vi "Set_TempHumWindDir_Calibration.vi"(5 "Wind dir off":i32, 6 "Path":path, 7 "Outside hum":dbl, 8 "Inside hum.":dbl, 9 "Outside temp":dbl min=-7.0 max=7.0 step=0.01, 10 "Inside temp":dbl min=-7.0 max=7.0 step=0.01) -> (0 "Cor. out hum":dbl, 1 "Cor. in hum":dbl, 2 "Cor. out temp":dbl, 3 "Cor. in temp":dbl, 4 "Calibration values set?":bool)   [LabVIEW 2012]
uses:
  VantagePro.dll
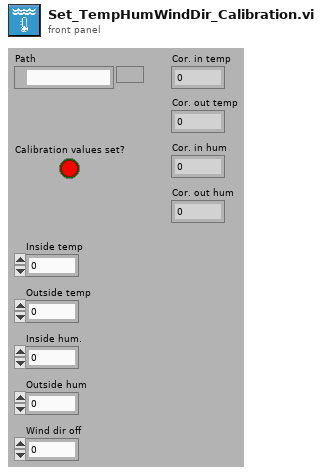
[diagram p1: front panel]
types:
  T1 = cluster{"In Temp":sgl, "Out Temp":sgl, "In Hum":u8, "Out Hum":u8, "Dum":i8, "Dum":i8, "Off In Temp":sgl, "Off Out Temp":sgl, "Off In Hum":i8, "Off Out Hum":i8}
  T2 = cluster{"In Temp":dbl, "Out Temp":dbl, "In Hum":dbl, "Out Hum":dbl}
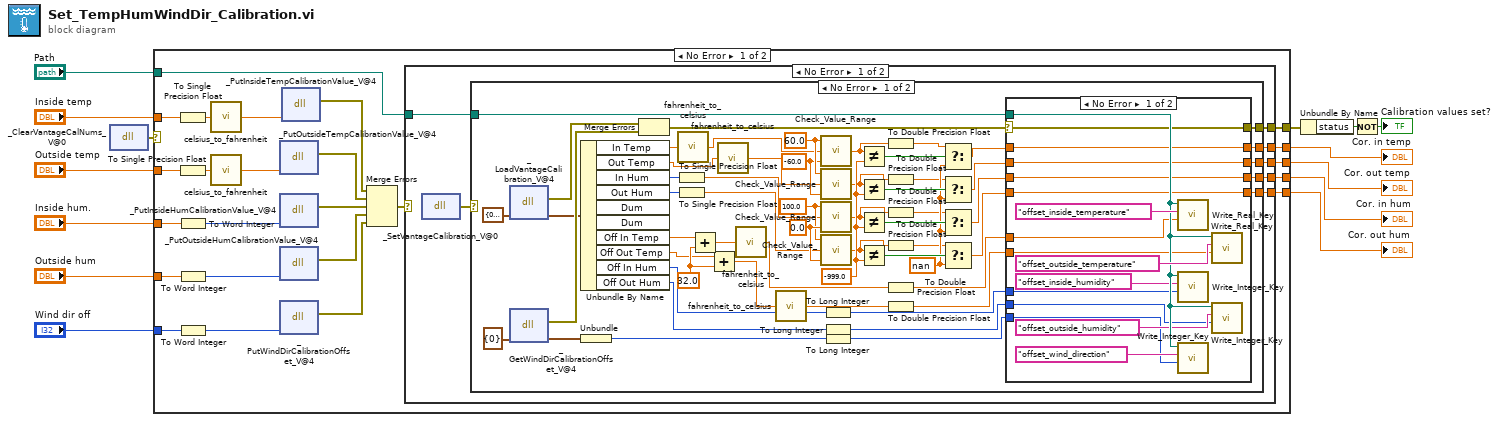
[diagram p0: block diagram]
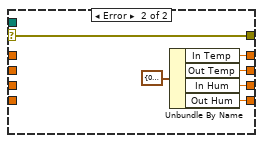
[diagram p2: hidden frame]
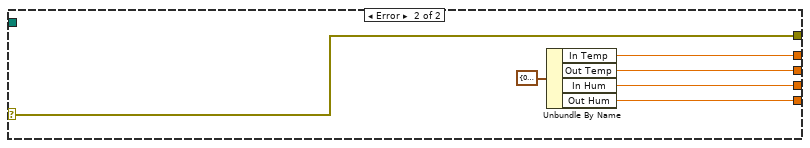
[diagram p3: hidden frame]
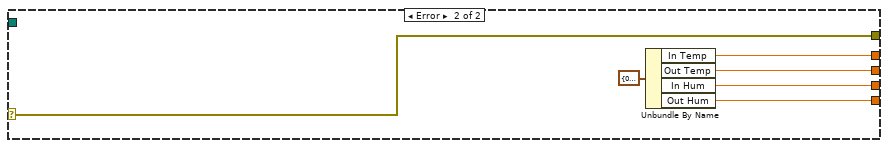
[diagram p4: hidden frame]
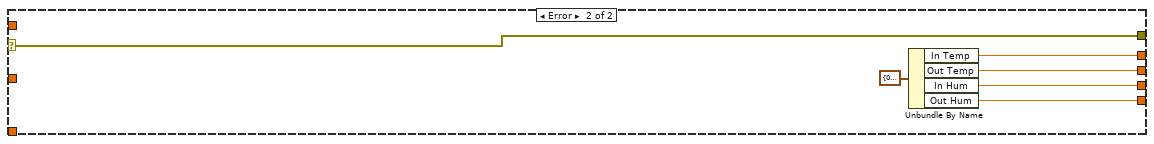
[diagram p5: hidden frame]
diagram:
  n1 = dll-call lib="C:/Users/Bob van Eijk/Desktop/LabView Projects 12/HiSPARC Weather Station/VantagePro.dll" fn="_ClearVantageCalNums_V@0" label="Clear Cal Nums"() -> (error out=w14:errorcluster)  [unwired: 4 in, 1 out]
  n2 = case shown="No Error" w14 {
    selector: w14 -> [_ w143]
    tunnel: "Inside temp" -> [w27 _]
    tunnel: "Inside hum." -> [w25 _]
    tunnel: "Outside temp" -> [w26 _]
    tunnel: "Outside hum" -> [w24 _]
    tunnel: "Wind dir off" -> [w23 _]
    tunnel: "Path" -> [w33 _]
    tunnel: [w32 w143] -> w7
    tunnel: [w31 w141] -> w4
    tunnel: [w30 w140] -> w3
    tunnel: [w29 w139] -> w2
    tunnel: [w28 w138] -> w1
    frame No Error {
      n3 = To Single Precision Float(number=w27) -> (single precision float=w35:sgl)
      n4 = To Single Precision Float(number=w26) -> (single precision float=w36:sgl)
      n5 = To Word Integer(number=w25) -> (16bit integer=w16:i16)
      n6 = To Word Integer(number=w24) -> (16bit integer=w15:i16)
      n7 = To Word Integer(number=w23) -> (16bit integer=w37:i16)
      n8 = call "celsius_to_fahrenheit.vi"("Celcius"=w35) -> ("Fahrenheit"=w22:sgl)
      n9 = call "celsius_to_fahrenheit.vi"("Celcius"=w36) -> ("Fahrenheit"=w17:sgl)
      n10 = dll-call lib="C:/Users/Bob van Eijk/Desktop/LabView Projects 12/HiSPARC Weather Station/VantagePro.dll" fn="_PutOutsideTempCalibrationValue_V@4" label="Put Out Temp Cal Val"("valValue"=w17) -> (error out=w20:errorcluster)  [unwired: 5 in, 1 out]
      n11 = dll-call lib="C:/Users/Bob van Eijk/Desktop/LabView Projects 12/HiSPARC Weather Station/VantagePro.dll" fn="_PutInsideHumCalibrationValue_V@4" label="Put In Hum Cal Val"("calValue"=w16) -> (error out=w19:errorcluster)  [unwired: 5 in, 1 out]
      n12 = dll-call lib="C:/Users/Bob van Eijk/Desktop/LabView Projects 12/HiSPARC Weather Station/VantagePro.dll" fn="_PutOutsideHumCalibrationValue_V@4" label="Put Out Hum Cal Val"("calValue"=w15) -> (error out=w18:errorcluster)  [unwired: 5 in, 1 out]
      n13 = dll-call lib="C:/Users/Bob van Eijk/Desktop/LabView Projects 12/HiSPARC Weather Station/VantagePro.dll" fn="_PutWindDirCalibrationOffset_V@4" label="Wind dir Offset"("winddirectionoff"=w37) -> (error out=w38:errorcluster)  [unwired: 5 in, 1 out]
      n14 = dll-call lib="C:/Users/Bob van Eijk/Desktop/LabView Projects 12/HiSPARC Weather Station/VantagePro.dll" fn="_PutInsideTempCalibrationValue_V@4" label="Put In Temp Cal Val"("calValue"=w22) -> (error out=w21:errorcluster)  [unwired: 5 in, 1 out]
      n15 = Merge Errors(w21, w20, w19, w18, w38) -> (w34:errorcluster)
      n16 = case shown="No Error" w34 {
        selector: w34 -> [_ w137]
        tunnel: [w43 w137] -> w32
        tunnel: w33 -> [w44 _]
        tunnel: [w42 w135] -> w31
        tunnel: [w41 w134] -> w30
        tunnel: [w40 w133] -> w29
        tunnel: [w39 w132] -> w28
        frame No Error {
          n17 = dll-call lib="C:/Users/Bob van Eijk/Desktop/LabView Projects 12/HiSPARC Weather Station/VantagePro.dll" fn="_SetVantageCalibration_V@0" label="Set cal. val."() -> (error out=w45:errorcluster)  [unwired: 4 in, 1 out]
          n18 = case shown="No Error" w45 {
            selector: w45 -> [_ w126]
            tunnel: [w81 w127] -> w39
            tunnel: [w82 w128] -> w40
            tunnel: [w83 w129] -> w41
            tunnel: [w84 w130] -> w42
            tunnel: [w79 w126] -> w43
            tunnel: w44 -> [w80 _]
            frame No Error {
              w59 = nan ("Data_input")
              w68 = sgl -999.0 ("Min")
              w78 = sgl 0.0 ("Min")
              w77 = sgl 100.0 ("Max")
              w75 = sgl -60.0 ("Min")
              w76 = sgl 60.0 ("Max")
              w96 = sgl 32.0
              n19 = dll-call lib="C:/Users/Bob van Eijk/Desktop/LabView Projects 12/HiSPARC Weather Station/VantagePro.dll" fn="_LoadVantageCalibration_V@4" label="Temp&hum data"("calibration"=T1 {"In Temp"=0.0, "Out Temp"=0.0, "In Hum"=0, "Out Hum"=0, "Dum"=0, "Dum"=0, "Off In Temp"=0.0, "Off Out Temp"=0.0, "Off In Hum"=0, "Off Out Hum"=0}) -> (error out=w100:errorcluster, "calibration"=w93:T1)  [unwired: 4 in, 1 out]
              n20 = dll-call lib="C:/Users/Bob van Eijk/Desktop/LabView Projects 12/HiSPARC Weather Station/VantagePro.dll" fn="_GetWindDirCalibrationOffset_V@4" label="Wind dir offset"("winddirectionoff"=cluster{i32} {0}) -> (error out=w101:errorcluster, "winddirectionoff"=w103:cluster{i32})  [unwired: 4 in, 1 out]
              n21 = Unbundle By Name(w93) -> ("In Temp"=w99:sgl, "Out Temp"=w91:sgl, "In Hum"=w72:u8, "Out Hum"=w71:u8, "Off In Temp"=w92:sgl, "Off Out Temp"=w95:sgl, "Off In Hum"=w88:i8, "Off Out Hum"=w87:i8)  [unwired: 2 out]
              n22 = Unbundle(w103) -> (w86:i32)
              n23 = Merge Errors(w100, w101) -> (w85:errorcluster)
              n24 = To Single Precision Float(number=w72) -> (single precision float=w70:sgl)
              n25 = To Single Precision Float(number=w71) -> (single precision float=w69:sgl)
              n26 = call "fahrenheit_to_celsius.vi"("Fahrenheit"=w99) -> ("Celsius"=w74:sgl)
              n27 = Add(x=w92, y=w96) -> (x+y=w97:sgl)
              n28 = Add(x=w95, y=w96) -> (x+y=w98:sgl)
              n29 = call "fahrenheit_to_celsius.vi"("Fahrenheit"=w91) -> ("Celsius"=w73:sgl)
              n30 = call "fahrenheit_to_celsius.vi"("Fahrenheit"=w97) -> ("Celsius"=w90:sgl)
              n31 = call "fahrenheit_to_celsius.vi"("Fahrenheit"=w98) -> ("Celsius"=w89:sgl)
              n32 = call "Check_Value_Range.vi"("Min"=w75, "Data in"=w74, "Max"=w76) -> ("Data out"=w63:sgl)
              n33 = call "Check_Value_Range.vi"("Min"=w75, "Data in"=w73, "Max"=w76) -> ("Data out"=w62:sgl)
              n34 = call "Check_Value_Range.vi"("Min"=w78, "Data in"=w70, "Max"=w77) -> ("Data out"=w61:sgl)
              n35 = call "Check_Value_Range.vi"("Min"=w78, "Data in"=w69, "Max"=w77) -> ("Data out"=w60:sgl)
              n36 = To Long Integer(number=w88) -> (32bit integer=w54:i32)
              n37 = To Long Integer(number=w87) -> (32bit integer=w53:i32)
              n38 = To Long Integer(number=w86) -> (32bit integer=w52:i32)
              n39 = Not Equal?(x=w63, y=w68) -> (x != y?=w67:bool)
              n40 = Not Equal?(x=w62, y=w68) -> (x != y?=w65:bool)
              n41 = Not Equal?(x=w61, y=w68) -> (x != y?=w64:bool)
              n42 = Not Equal?(x=w60, y=w68) -> (x != y?=w66:bool)
              n43 = To Double Precision Float(number=w63) -> (double precision float=w49:dbl)
              n44 = To Double Precision Float(number=w62) -> (double precision float=w48:dbl)
              n45 = To Double Precision Float(number=w61) -> (double precision float=w47:dbl)
              n46 = To Double Precision Float(number=w60) -> (double precision float=w46:dbl)
              n47 = To Double Precision Float(number=w90) -> (double precision float=w51:dbl)
              n48 = To Double Precision Float(number=w89) -> (double precision float=w50:dbl)
              n49 = Select(t=w49, s=w67, f=w59) -> (s? t:f=w58:dbl)
              n50 = Select(t=w48, s=w65, f=w59) -> (s? t:f=w57:dbl)
              n51 = Select(t=w47, s=w64, f=w59) -> (s? t:f=w56:dbl)
              n52 = Select(t=w46, s=w66, f=w59) -> (s? t:f=w55:dbl)
              n53 = case shown="No Error" w85 {
                selector: w85 -> [w113 w125]
                tunnel: w58 -> [w107 _]
                tunnel: w57 -> [w106 _]
                tunnel: w56 -> [w105 _]
                tunnel: w55 -> [w104 _]
                tunnel: w51 -> [w112 _]
                tunnel: w50 -> [w111 _]
                tunnel: w54 -> [w110 _]
                tunnel: w53 -> [w109 _]
                tunnel: w52 -> [w108 _]
                tunnel: [w107 w123] -> w84
                tunnel: [w106 w122] -> w83
                tunnel: [w105 w121] -> w82
                tunnel: [w104 w120] -> w81
                tunnel: w80 -> [w116 _]
                tunnel: [w113 w125] -> w79
                frame No Error {
                  n54 = call "Write_Real_Key.vi"("Key value"=w112, "Key name"="offset_inside_temperature" ("key"), "Configuration file path"=w116) -> ()  [unwired: 2 in, 3 out]
                  n55 = call "Write_Integer_Key.vi"("Key value"=w110, "Key name"="offset_inside_humidity" ("key"), "Configuration file path"=w116) -> ()  [unwired: 2 in, 3 out]
                  n56 = call "Write_Integer_Key.vi"("Key value"=w108, "Key name"="offset_wind_direction" ("key"), "Configuration file path"=w116) -> ()  [unwired: 2 in, 3 out]
                  n57 = call "Write_Real_Key.vi"("Key value"=w111, "Key name"="offset_outside_temperature" ("key"), "Configuration file path"=w116) -> ()  [unwired: 2 in, 3 out]
                  n58 = call "Write_Integer_Key.vi"("Key value"=w109, "Key name"="offset_outside_humidity" ("key"), "Configuration file path"=w116) -> ()  [unwired: 2 in, 3 out]
                }
                frame Error {
                  n59 = Unbundle By Name(T2 {"In Temp"=0.0, "Out Temp"=0.0, "In Hum"=0.0, "Out Hum"=0.0}) -> ("In Temp"=w123:dbl, "Out Temp"=w122:dbl, "In Hum"=w121:dbl, "Out Hum"=w120:dbl)
                }
              }
            }
            frame Error {
              n60 = Unbundle By Name(T2 {"In Temp"=0.0, "Out Temp"=0.0, "In Hum"=0.0, "Out Hum"=0.0}) -> ("In Temp"=w130:dbl, "Out Temp"=w129:dbl, "In Hum"=w128:dbl, "Out Hum"=w127:dbl)
            }
          }
        }
        frame Error {
          n61 = Unbundle By Name(T2 {"In Temp"=0.0, "Out Temp"=0.0, "In Hum"=0.0, "Out Hum"=0.0}) -> ("In Temp"=w135:dbl, "Out Temp"=w134:dbl, "In Hum"=w133:dbl, "Out Hum"=w132:dbl)
        }
      }
    }
    frame Error {
      n62 = Unbundle By Name(T2 {"In Temp"=0.0, "Out Temp"=0.0, "In Hum"=0.0, "Out Hum"=0.0}) -> ("In Temp"=w141:dbl, "Out Temp"=w140:dbl, "In Hum"=w139:dbl, "Out Hum"=w138:dbl)
    }
  }
  "Cor. in temp" <- w4
  "Cor. out temp" <- w3
  "Cor. in hum" <- w2
  "Cor. out hum" <- w1
  n63 = Unbundle By Name(w7) -> ("status"=w6:bool)
  n64 = Not(x=w6) -> (.not. x?=→"Calibration values set?":bool)
